vi "Get_ADAM_averages_client.vi"(6 "No of averages":i32=1, 7 "All Active Channels":bool, 9 "End time":dbl, 10 "Start time":dbl, 11 "ADAM Ch Names":string[](array[string])) -> (1 "Values":string[][](array[string]), 2 "Comments":string[](array[string]), 3 "Titles":string[](array[string]), 4 "Messages":string, 5 "DBL values":dbl[][](array[numeric]) format="%.2f")   [LabVIEW 2020]
doc: "This is an example of using features of the VI Server as a client. It shows how you might browse from one or more applications that may be exporting data from one or more data stations. \n\nThe example shows how to query a server for its list of exported VIs, how to get references to the VIs, and how call them with the Call By Reference function."
uses:
  Anemometry/Anemometry Sub Vis/Controls/Global_mode.ctl
  Sub VIs/ADAM Controls/Channel_names.ctl
  Anemometry/Anemometry Sub Vis/Globals/Preference_global.vi
panel:
  in  "vi type":refnum<vi>
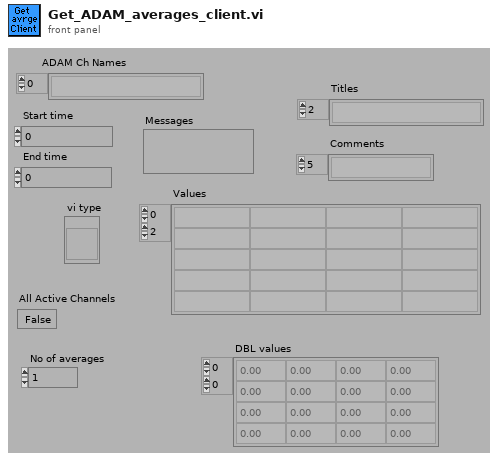
[diagram p1: front panel]
types:
  T1 = typedef "Global_mode.ctl" = enum16{"Read Global", "Load Global From File", "Write Global to File"}
  T2 = typedef "Channel_names.ctl" = enum16{"Active Only", "Active + Off", "All Channels"}
  T3 = typedef "Server_Comms.ctl" = enum16{"Do Not Link To Server", "Server Link Healthy"}
  T4 = typedef "Update_scan_value.ctl" = cluster{"Channel Name":string, "New Value":dbl}
  T5 = typedef "Ch_description_ADAM.ctl" = cluster{"Ch Name":string, "Type":T6, "Function":T7, "Ch State":T8, "Calibration type":T9, "A":dbl, "B":dbl, "C":dbl, "D":dbl, "Comments":string, "Address":T10, "String":string, "Duty":u16}
  T6 = typedef "Module_type_ADAM.ctl" = string
  T7 = typedef "Function_ADAM.ctl" = enum16{"Analogue Input", "Digital Input", "Event counter", "Event rate", "Analogue Output", "Digital Output", "Relay Output"}
  T8 = typedef "Channel_State.ctl" = enum16{"On", "Off", "Always On", "Always Off"}
  T9 = typedef "Calib_type_ADAM.ctl" = string
  T10 = typedef "Address.ctl" = cluster{"Main":i32, "Ch.":i32, "Sub":i32, "Port Name":string}
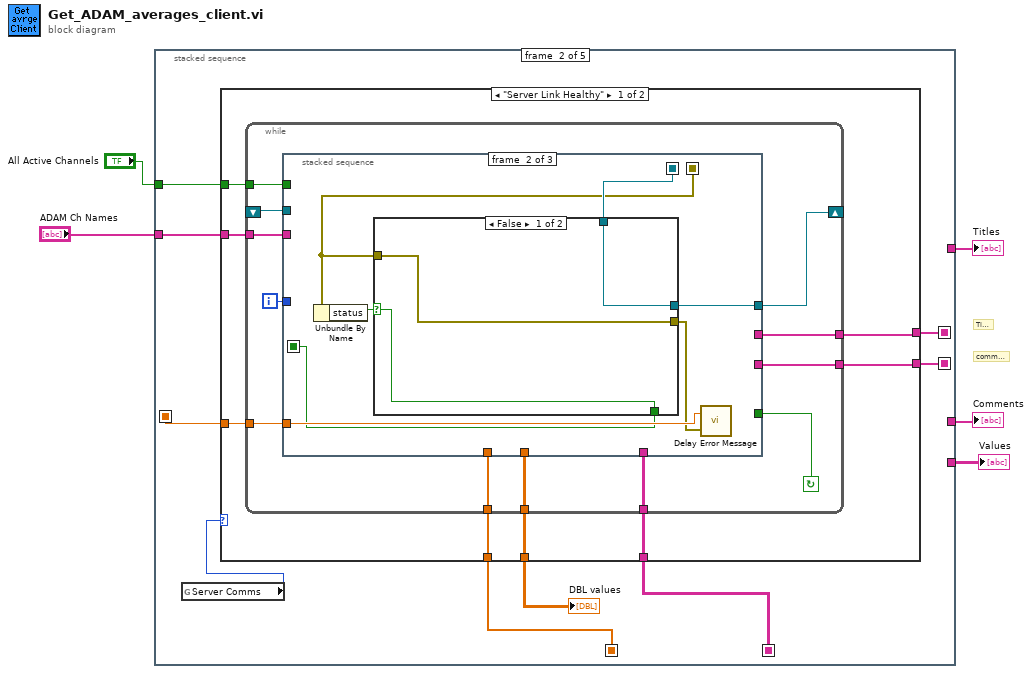
[diagram p0: block diagram]
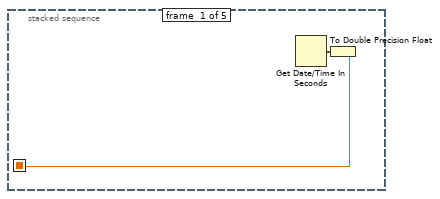
[diagram p2: hidden frame]
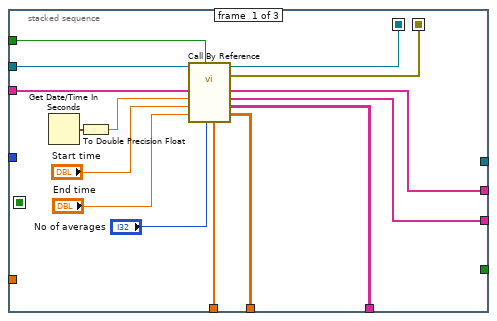
[diagram p3: hidden frame]
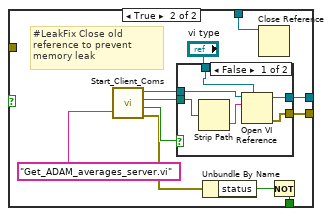
[diagram p4: hidden frame]
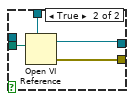
[diagram p5: hidden frame]
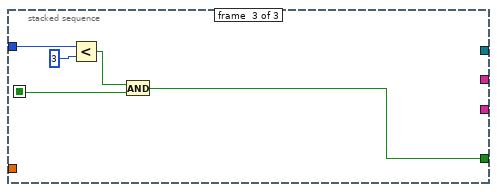
[diagram p6: hidden frame]
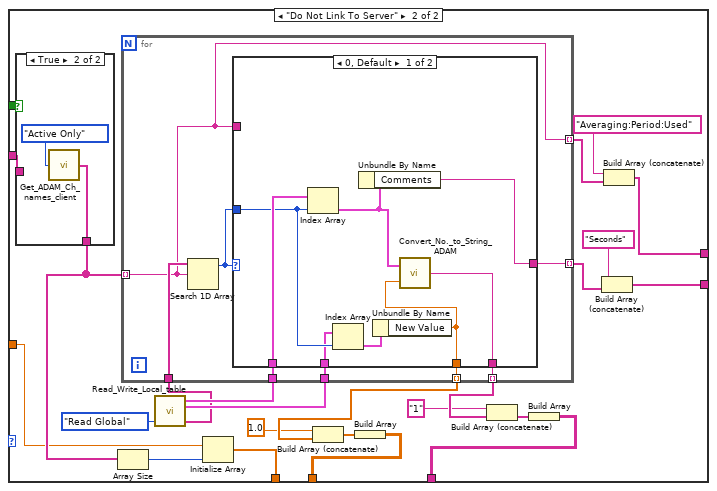
[diagram p7: hidden frame]
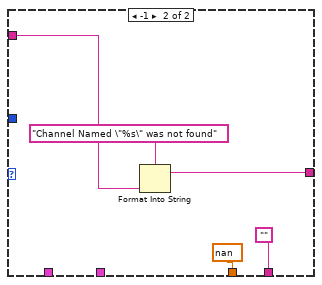
[diagram p9: hidden frame]
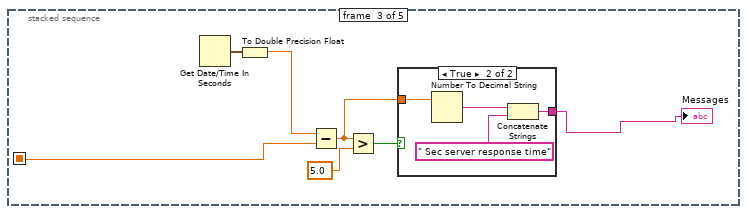
[diagram p10: hidden frame]
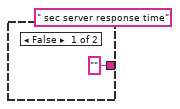
[diagram p11: hidden frame]
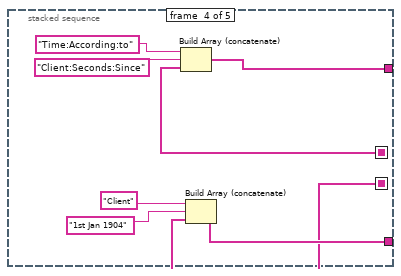
[diagram p12: hidden frame]
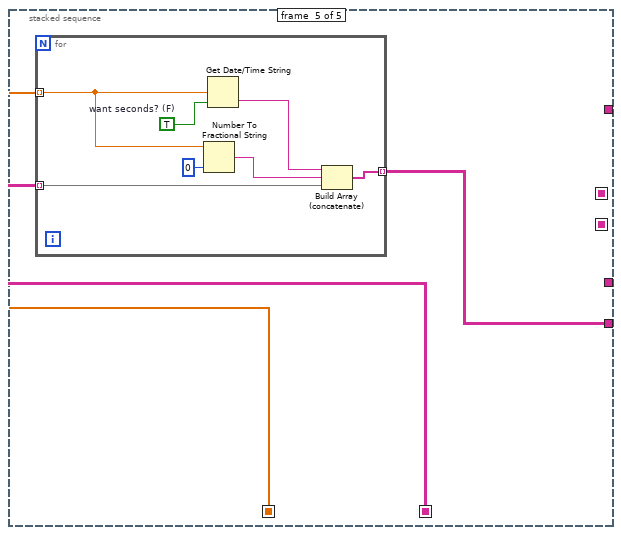
[diagram p13: hidden frame]
diagram:
  # "comments"
  # "Titles"
  n1 = stacked-sequence {
    seq-local: [_ w16 _ _ _] -> [_ _ _ w155 _]
    seq-local: [_ w8 _ _ _] -> [_ _ _ w148 _]
    seq-local: [_ w15 _ _ _] -> [_ _ _ _ w157]
    seq-local: [w7 _ _ _ _] -> [_ w14 w141 _ _]
    seq-local: [_ w13 _ _ _] -> [_ _ _ _ w158]
    tunnel: [_ _ _ w153 _] -> w5
    tunnel: [_ _ _ w154 _] -> w4
    tunnel: [_ _ _ _ w156] -> w3
    tunnel: "ADAM Ch Names" -> [_ w10 _ _ _]
    tunnel: "All Active Channels" -> [_ w9 _ _ _]
    frame #0 {
      n2 = Get Date/Time In Seconds() -> (seconds since 1Jan1904=w6:timestamp)
      n3 = To Double Precision Float(number=w6) -> (double precision float=w7:dbl)
    }
    frame #1 {
      n4 = global read "Preference_global.vi" "Server Comms"() -> (w12:T3)
      n5 = case shown="\"Server Link Healthy\"" w12 {
        tunnel: [w24 w94] -> w16
        tunnel: [w23 w102] -> w15
        tunnel: w14 -> [w22 w92]
        tunnel: [w21 w107] -> w13
        tunnel: [w20 w88] -> w11
        tunnel: w10 -> [w19 w103]
        tunnel: w9 -> [w18 w106]
        tunnel: [w17 w93] -> w8
        frame "Server Link Healthy" {
          n6 = while {
            shift-left: _ -> [w31]
            shift-right: [w30] -> _
            tunnel: [w32] -> w21
            tunnel: w22 -> [w33]
            tunnel: [w34] -> w23
            tunnel: [w35] -> w17
            tunnel: [w36] -> w24
            tunnel: [w27] -> w20
            tunnel: w19 -> [w26]
            tunnel: w18 -> [w25]
            i -> [w29]
            stop <- w28 continue-if-true
            n7 = stacked-sequence {
              seq-local: [w41 _ _] -> [_ w57 _]
              seq-local: [w42 _ _] -> [_ w55 _]
              seq-local: [_ w52 _] -> [_ _ w84]
              tunnel: [w44 _ _] -> w36
              tunnel: [w49 _ _] -> w35
              tunnel: [w48 _ _] -> w34
              tunnel: w33 -> [_ w54 _]
              tunnel: [w46 _ _] -> w32
              tunnel: w31 -> [w43 _ _]
              tunnel: [_ w58 _] -> w30
              tunnel: w29 -> [_ _ w85]
              tunnel: [_ _ w83] -> w28
              tunnel: [w39 _ _] -> w27
              tunnel: w26 -> [w38 _ _]
              tunnel: w25 -> [w37 _ _]
              frame #0 {
                n8 = Get Date/Time In Seconds() -> (seconds since 1Jan1904=w40:timestamp)
                n9 = To Double Precision Float(number=w40) -> (double precision float=w50:dbl)
                n10 = call-by-ref "?"(reference=w43, "No of averages"="No of averages", "All Active Channels"=w37, "End time"="End time", "Start time"="Start time", "Clients time"=w50, "ADAM Ch Names"=w38) -> (reference out=w41:refnum<vi>, error out=w42:errorcluster, "DBL values"=w39:dbl[][], "Values"=w48:string[][], "Comments"=w49:string[], "Titles"=w44:string[], "Times"=w46:dbl[])  [unwired: 1 in]
              }
              frame #1 {
                n11 = Unbundle By Name(w55) -> ("status"=w56:bool)
                n12 = case shown="False" w56 {
                  selector: w56 -> [w59 _]
                  tunnel: [w61 w68] -> w58
                  tunnel: w57 -> [w61 w65]
                  tunnel: [w60 w66] -> w53
                  tunnel: w55 -> [w60 _]
                  tunnel: [w59 w62] -> w52
                  frame False {
                  }
                  frame True {
                    # "#LeakFix Close old reference to prevent memory leak"
                    n13 = call "Start_Client_Coms.vi"("VI name to run on server"="Get_ADAM_averages_server.vi") -> ("LabVIEW application reference"=w70:refnum<vi>, "Checked VI name"=w71:path, "Local Call"=w69:bool, "Error cluster"=w63:errorcluster)  [unwired: 1 in]
                    n14 = case shown="False" w69 {
                      tunnel: [w76 w82] -> w68
                      tunnel: "vi type" -> [w75 w81]
                      tunnel: w71 -> [w74 w80]
                      tunnel: w70 -> [w73 _]
                      tunnel: [w77 w79] -> w66
                      frame False {
                        n15 = Strip Path(path=w74) -> (name=w78:string)  [unwired: 1 out]
                        n16 = Open VI Reference(type specifier VI Refnum (for type only)=w75, application reference (local)=w73, vi path=w78) -> (vi reference=w76:refnum<vi>, error out=w77:errorcluster)  [unwired: 1 in, 2 out]
                      }
                      frame True {
                        n17 = Open VI Reference(type specifier VI Refnum (for type only)=w81, vi path=w80) -> (vi reference=w82:refnum<vi>, error out=w79:errorcluster)  [unwired: 1 in, 3 out]
                      }
                    }
                    n18 = Unbundle By Name(w63) -> ("status"=w64:bool)
                    n19 = Close Reference(reference=w65) -> ()  [unwired: 1 in, 1 out]
                    n20 = Not(x=w64) -> (.not. x?=w62:bool)
                  }
                }
                n21 = call "Delay Error Message.vi"("error in (no error)"=w53, "Seconds since 1904"=w54) -> ()  [unwired: 2 in]
              }
              frame #2 {
                n22 = Less?(x=w85, y=3) -> (x < y?=w86:bool)
                n23 = And(x=w86, y=w84) -> (x .and. y?=w83:bool)
              }
            }
          }
        }
        frame "Do Not Link To Server" {
          n24 = case shown="True" w106 {
            tunnel: [w112 w113] -> w105
            tunnel: w103 -> [w112 _]
            frame False {
            }
            frame True {
              n25 = call "Get_ADAM_Ch_names_client.vi"("Channel names set"=Channel_names."Active Only") -> ("Ch names"=w113:string[])
            }
          }
          n26 = Array Size(array=w105) -> (size(s)=w108:i32)
          n27 = call "Read_Write_Local_table.vi"("Mode"=Global_mode."Read Global") -> ("Ch Names"=w104:string[], "Ch Values Out"=w109:T4[], "Channels Descriptions Out"=w110:T5[])  [unwired: 2 in]
          n28 = for {
            tunnel: w104 -> [w119]
            tunnel: w105 -> [w118] mode=indexing
            tunnel: w110 -> [w121]
            tunnel: w109 -> [w120]
            tunnel: [w118] -> w95 mode=indexing
            tunnel: [w117] -> w99 mode=indexing
            tunnel: [w116] -> w101 mode=indexing
            tunnel: [w115] -> w91 mode=indexing
            n29 = Search 1D Array(1D array=w119, element=w118) -> (index of element=w122:i32)  [unwired: 1 out]
            n30 = case shown="0, Default" w122 {
              tunnel: w122 -> [w129 _]
              tunnel: w121 -> [w130 _]
              tunnel: w120 -> [w128 _]
              tunnel: w118 -> [_ w135]
              tunnel: [w125 w133] -> w117
              tunnel: [w124 ""] -> w116
              tunnel: [w123 nan ("New Value")] -> w115
              frame 0, Default {
                n31 = Index Array(array=w130, index=w129) -> (element=w126:T5)
                n32 = Index Array(array=w128, index=w129) -> (element=w127:T4)
                n33 = Unbundle By Name(w126) -> ("Comments"=w125:string)
                n34 = Unbundle By Name(w127) -> ("New Value"=w123:dbl)
                n35 = call "Convert_No._to_String_ADAM.vi"("Input number"=w123, "Ch Description"=w126) -> ("Output sting"=w124:string)
              }
              frame -1 {
                n36 = Format Into String(format string="Channel Named \"%s\" was not found" ("Format String"), w135) -> (resulting string=w133:string)  [unwired: 2 in, 1 out]
              }
            }
          }
          n37 = Initialize Array(w92, w108) -> (w107:dbl[])
          n38 = Build Array (concatenate)(1.0, w91) -> (w89:dbl[])
          n39 = Build Array(w89) -> (w88:dbl[][])
          n40 = Build Array (concatenate)("1", w101) -> (w100:string[])
          n41 = Build Array(w100) -> (w102:string[][])
          n42 = Build Array (concatenate)("Seconds", w99) -> (w93:string[])
          n43 = Build Array (concatenate)("Averaging:Period:Used", w95) -> (w94:string[])
        }
      }
      "DBL values" <- w11
    }
    frame #2 {
      n44 = Get Date/Time In Seconds() -> (seconds since 1Jan1904=w137:timestamp)
      n45 = To Double Precision Float(number=w137) -> (double precision float=w142:dbl)
      n46 = Subtract(x=w142, y=w141) -> (x-y=w138:dbl)
      n47 = Greater?(x=w138, y=5.0) -> (0:w139:bool)
      n48 = case shown="True" w139 {
        tunnel: w138 -> [_ w147]
        tunnel: ["" w144] -> w136
        frame False {
          (unwired) " sec server response time"
        }
        frame True {
          n49 = Number To Decimal String(number=w147) -> (decimal integer string=w145:string)  [unwired: 1 out]
          n50 = Concatenate Strings(w145, " Sec server response time") -> (w144:string)
        }
      }
      "Messages" <- w136
    }
    frame #3 {
      n51 = Build Array (concatenate)("Time:According:to", "Client:Seconds:Since", w155) -> (w153:string[])
      n52 = Build Array (concatenate)("Client" ("Comments"), "1st Jan 1904" ("Comments"), w148) -> (w154:string[])
    }
    frame #4 {
      n53 = for {
        tunnel: w158 -> [w160] mode=indexing
        tunnel: [w165] -> w156 mode=indexing
        tunnel: w157 -> [w164] mode=indexing
        w163 = TRUE  # want seconds? (F)
        n54 = Number To Fractional String(number=w160, precision (6)=i16 0) -> (F-format string=w159:string)  [unwired: 2 out]
        n55 = Get Date/Time String(seconds (now)=w160, want seconds? (F)=w163) -> (time string=w162:string)  [unwired: 2 out]
        n56 = Build Array (concatenate)(w162, w159, w164) -> (w165:string[])
      }
    }
  }
  "Titles" <- w5
  "Comments" <- w4
  "Values" <- w3
